vi "Eval.vi"(10 "String":string="1 + 1", 11 "NameSpace":variant) -> (3 "element":dbl)   [LabVIEW 2019, in "Eval.lvlib"]
uses:
  Library/Eval.lvlib
  <vilib>/Utility/Data Type/NI_Data Type.lvlib
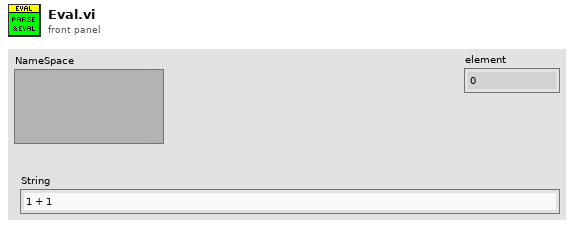
[diagram p1: front panel]
types:
  T1 = cluster{"Token":enum16{"ADD", "BITAND", "BITOR", "COMMA", "DIV", "Dnumeric", "EQUAL", "EXP", "FUNC", "GREATER", "GREATEREQ", "INumeric", "Identifier", "Ignore", "LESS", "LESSEQ", "LOGAND", "LOGOR", "LPAR", "LSHIFT", "MULT", "N/A", "RPAR", "RSHIFT", "SUB", "UADD", "USUB"}, "Priority":i32, "Type":enum16{"N/A", "GroupL", "GroupR", "Comma", "Operator", "Operand", "End"}, "Associtivity":enum16{"N/A", "L-R", "R-L"}, "GroupPair":i32}[]
  T2 = cluster{"NextTable":enum16{"#Init", "And", "Bin", "CompG", "CompL", "DNumeric", "INumeric", "Identifier", "Or", "Unreachable"}, "Actions":enum16{"Drop", "Hold", "Push"}, "Token":enum16{"ADD", "BITAND", "BITOR", "COMMA", "DIV", "Dnumeric", "EQUAL", "EXP", "FUNC", "GREATER", "GREATEREQ", "INumeric", "Identifier", "Ignore", "LESS", "LESSEQ", "LOGAND", "LOGOR", "LPAR", "LSHIFT", "MULT", "N/A", "RPAR", "RSHIFT", "SUB", "UADD", "USUB"}}[]
  T3 = cluster{"NextTable":enum16{"#Init", "And", "Bin", "CompG", "CompL", "DNumeric", "INumeric", "Identifier", "Or", "Unreachable"}, "Actions":enum16{"Drop", "Hold", "Push"}, "Token":enum16{"ADD", "BITAND", "BITOR", "COMMA", "DIV", "Dnumeric", "EQUAL", "EXP", "FUNC", "GREATER", "GREATEREQ", "INumeric", "Identifier", "Ignore", "LESS", "LESSEQ", "LOGAND", "LOGOR", "LPAR", "LSHIFT", "MULT", "N/A", "RPAR", "RSHIFT", "SUB", "UADD", "USUB"}}
  T4 = enum16{"ADD", "BITAND", "BITOR", "COMMA", "DIV", "Dnumeric", "EQUAL", "EXP", "FUNC", "GREATER", "GREATEREQ", "INumeric", "Identifier", "Ignore", "LESS", "LESSEQ", "LOGAND", "LOGOR", "LPAR", "LSHIFT", "MULT", "N/A", "RPAR", "RSHIFT", "SUB", "UADD", "USUB"}
  T5 = cluster{"Start":i32, "End":i32, "Token":enum16{"ADD", "BITAND", "BITOR", "COMMA", "DIV", "Dnumeric", "EQUAL", "EXP", "FUNC", "GREATER", "GREATEREQ", "INumeric", "Identifier", "Ignore", "LESS", "LESSEQ", "LOGAND", "LOGOR", "LPAR", "LSHIFT", "MULT", "N/A", "RPAR", "RSHIFT", "SUB", "UADD", "USUB"}}
  T6 = cluster{"Start":i32, "End":i32, "Token":enum16{"ADD", "BITAND", "BITOR", "COMMA", "DIV", "Dnumeric", "EQUAL", "EXP", "FUNC", "GREATER", "GREATEREQ", "INumeric", "Identifier", "Ignore", "LESS", "LESSEQ", "LOGAND", "LOGOR", "LPAR", "LSHIFT", "MULT", "N/A", "RPAR", "RSHIFT", "SUB", "UADD", "USUB"}}[]
  T7 = enum16{"#Init", "And", "Bin", "CompG", "CompL", "DNumeric", "INumeric", "Identifier", "Or", "Unreachable"}
  T8 = cluster{"Token":enum16{"ADD", "BITAND", "BITOR", "COMMA", "DIV", "Dnumeric", "EQUAL", "EXP", "FUNC", "GREATER", "GREATEREQ", "INumeric", "Identifier", "Ignore", "LESS", "LESSEQ", "LOGAND", "LOGOR", "LPAR", "LSHIFT", "MULT", "N/A", "RPAR", "RSHIFT", "SUB", "UADD", "USUB"}, "Priority":i32, "Type":enum16{"N/A", "GroupL", "GroupR", "Comma", "Operator", "Operand", "End"}, "Associtivity":enum16{"N/A", "L-R", "R-L"}, "GroupPair":i32}
  T9 = enum16{"N/A", "GroupL", "GroupR", "Comma", "Operator", "Operand", "End"}
  T10 = typedef "NI_Data Type.lvlib/Data Type.ctl" = enum8{"Invalid Type", "Void", "I8", "I16", "I32", "I64", "U8", "U16", "U32", "U64", "Single Float", "Double Float", "Extended Float", "Single Complex", "Double Complex", "Extended Complex", "Enum U8", "Enum U16", "Enum U32", "Enum U64", "Single Float With Unit", "Double Float With Unit", "Extended Float With Unit", "Single Complex with Unit", "Double Complex with Unit", "Extended Complex with Unit", "Boolean", "String", "Path", "Picture", "Tag", "Array", "Cluster", "Variant", "LV Variant", "Waveform", "Timestamp", "Digital Waveform", "Digital Data", "ExpressData", "Refnum", "External Data", "VI", "Poly VI", "LabVIEW Class Instance", "Fixed Point", "Set Collection", "Map Collection"}
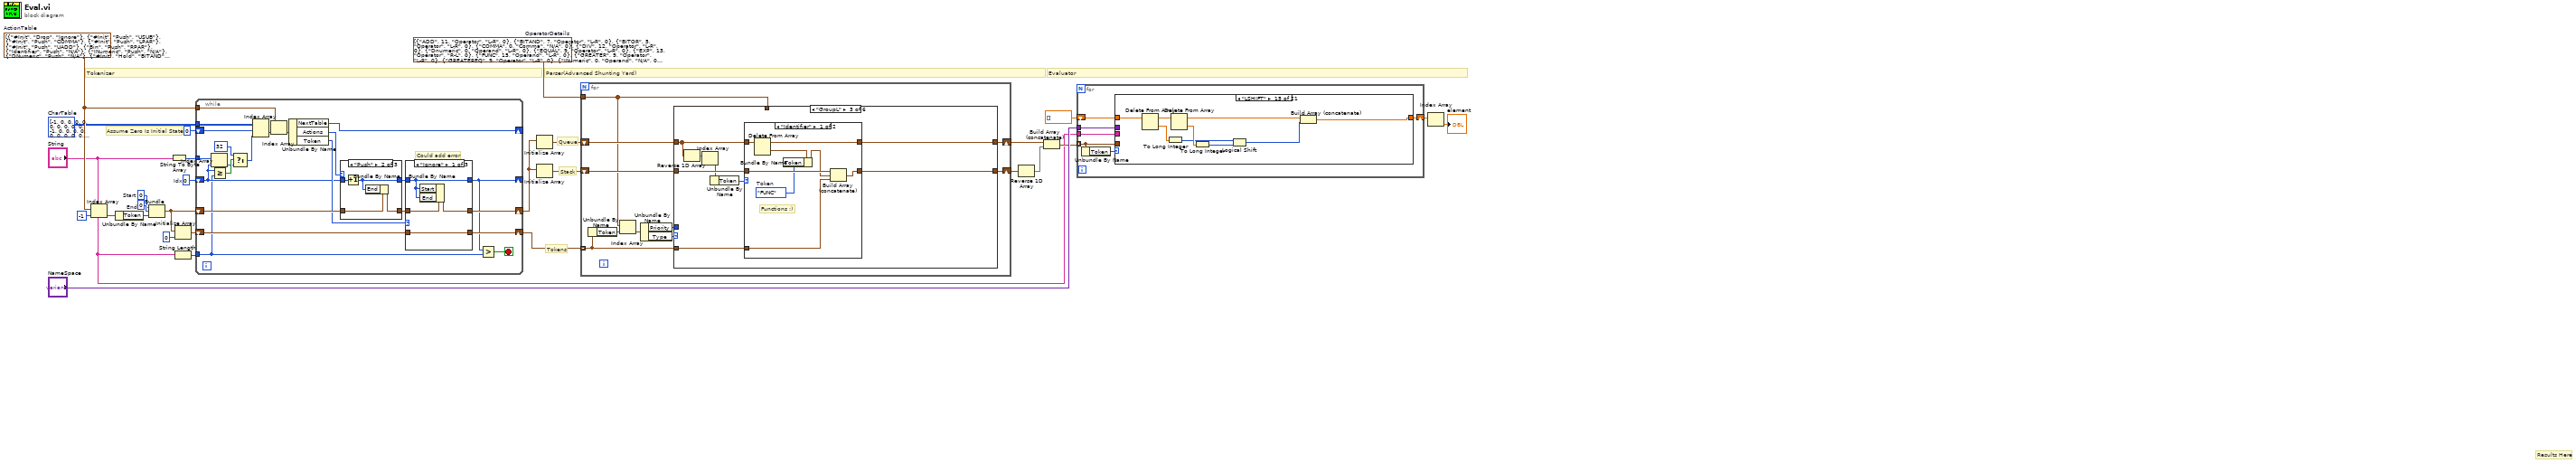
[diagram p0: block diagram]
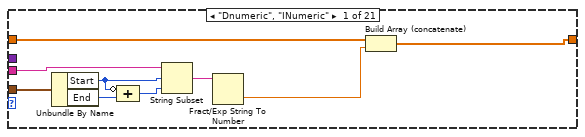
[diagram p2: hidden frame]
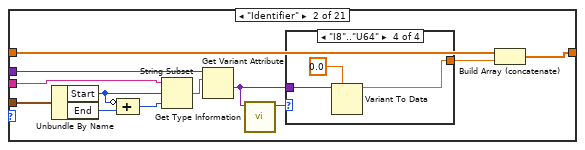
[diagram p3: hidden frame]
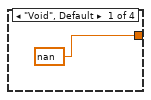
[diagram p4: hidden frame]
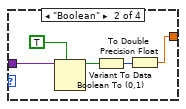
[diagram p5: hidden frame]
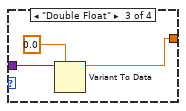
[diagram p6: hidden frame]
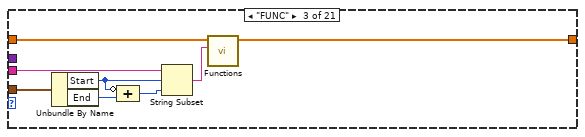
[diagram p7: hidden frame]
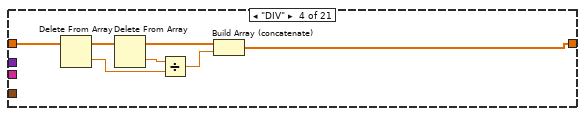
[diagram p8: hidden frame]
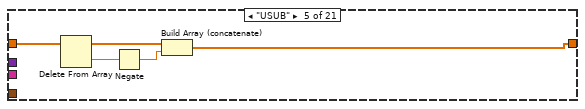
[diagram p9: hidden frame]
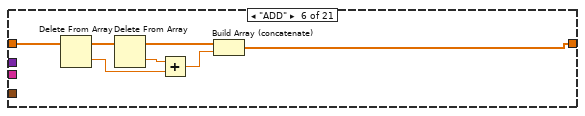
[diagram p10: hidden frame]
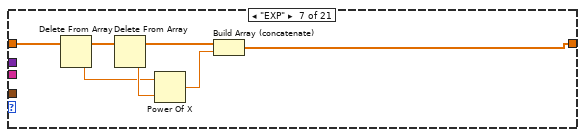
[diagram p11: hidden frame]
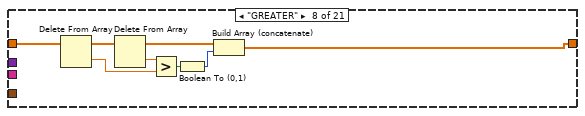
[diagram p12: hidden frame]
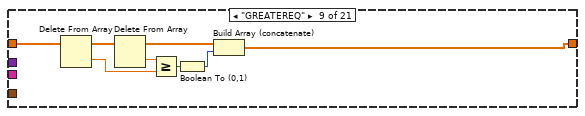
[diagram p13: hidden frame]
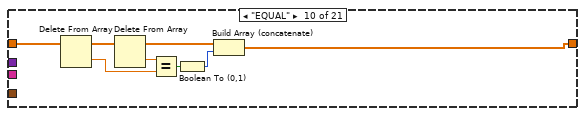
[diagram p14: hidden frame]
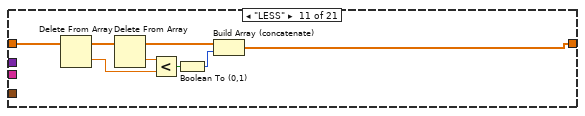
[diagram p15: hidden frame]
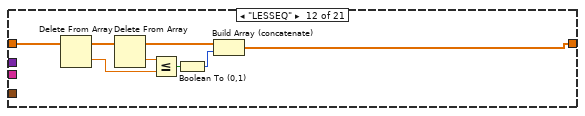
[diagram p16: hidden frame]
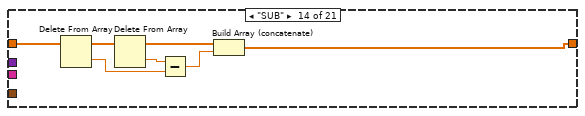
[diagram p18: hidden frame]
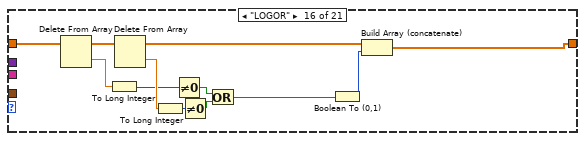
[diagram p19: hidden frame]
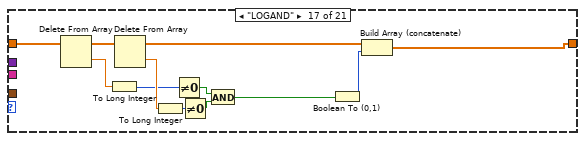
[diagram p20: hidden frame]
diagram:
  w3 = i32[][] [[-1, 0, 0, 0, 0, 0, 0, 0, 0, 0, -1, 0, 0, 0, 0, 0, 0, 0, 0, 0, 0, 0, 0, 0, 0, 0, 0, 0, 0, 0, 0, 0, 0, 0, 0, 0, 0, 0, 0, 0, 3, 5, 0, 4, 2, 1, 8, 0, 7, 7, 7, 7, 7, 7, 7, 7, 7, 7, 0, 0, 0, 0, 0, 0, 0, 6, 6, 6, 6, 6, 6, 6, 6, 6, 6, 6, 6, 6, 6, 6, 6, 6, 6, 6, 6, 6, 6, 6, 6, 6, 6, 0, 0, 0, 0, 6, 0, 6, 6, 6, 6, 6, 6, 6, 6, 6, 6, 6, 6, 6, 6, 6, 6, 6, 6, 6, 6, 6, 6, 6, 6, 6, 6, 0, 0, 0, 0, 0, 0, 0, 0, 0, 0, 0, 0, 0, 0, 0, 0, 0, 0, 0, 0, 0, 0, 0, 0, 0, 0, 0, 0, 0, 0, 0, 0, 0, 0, 0, 0, 0, 0, 0, 0, 0, 0, 0, 0, 0, 0, 0, 0, 0, 0, 0, 0, 0, 0, 0, 0, 0, 0, 0, 0, 0, 0, 0, 0, 0, 0, 0, 0, 0, 0, 0, 0, 0, 0, 0, 0, 0, 0, 0, 0, 0, 0, 0, 0, 0, 0, 0, 0, 0, 0, 0, 0, 0, 0, 0, 0, 0, 0, 0, 0, 0, 0, 0, 0, 0, 0, 0, 0, 0, 0, 0, 0, 0, 0, 0, 0, 0, 0, 0, 0, 0, 0, 0, 0, 0, 0, 0, 0, 0, 0, 0, 0], [-1, 9, 9, 9, 9, 9, 9, 9, 9, 9, -1, 9, 9, 9, 9, 9, 9, 9, 9, 9, 9, 9, 9, 9, 9, 9, 9, 9, 9, 9, 9, 9, 9, 9, 9, 9, 9, 9, 10, 9, 9, 9, 9, 9, 9, 9, 9, 9, 9, 9, 9, 9, 9, 9, 9, 9, 9, 9, 9, 9, 9, 9, 9, 9, 9, 9, 9, 9, 9, 9, 9, 9, 9, 9, 9, 9, 9, 9, 9, 9, 9, 9, 9, 9, 9, 9, 9, 9, 9, 9, 9, 9, 9, 9, 9, 9, 9, 9, 9, 9, 9, 9, 9, 9, 9, 9, 9, 9, 9, 9, 9, 9, 9, 9, 9, 9, 9, 9, 9, 9, 9, 9, 9, 9, 9, 9, 9, 9, 9, 9, 9, 9, 9, 9, 9, 9, 9, 9, 9, 9, 9, 9, 9, 9, 9, 9, 9, 9, 9, 9, 9, 9, 9, 9, 9, 9, 9, 9, 9, 9, 9, 9, 9, 9, 9, 9, 9, 9, 9, 9, 9, 9, 9, 9, 9, 9, 9, 9, 9, 9, 9, 9, 9, 9, 9, 9, 9, 9, 9, 9, 9, 9, 9, 9, 9, 9, 9, 9, 9, 9, 9, 9, 9, 9, 9, 9, 9, 9, 9, 9, 9, 9, 9, 9, 9, 9, 9, 9, 9, 9, 9, 9, 9, 9, 9, 9, 9, 9, 9, 9, 9, 9, 9, 9, 9, 9, 9, 9, 9, 9, 9, 9, 9, 9, 9, 9, 9, 9, 9, 9, 9, 9, 9, 9, 9], [-1, 11, 11, 11, 11, 11, 11, 11, 11, 11, -1, 11, 11, 11, 11, 11, 11, 11, 11, 11, 11, 11, 11, 11, 11, 11, 11, 11, 11, 11, 11, 11, 11, 11, 11, 11, 11, 11, 24, 11, 16, 20, 15, 17, 14, 13, 27, 12, 26, 26, 26, 26, 26, 26, 26, 26, 26, 26, 11, 11, 22, 18, 21, 11, 11, 25, 25, 25, 25, 25, 25, 25, 25, 25, 25, 25, 25, 25, 25, 25, 25, 25, 25, 25, 25, 25, 25, 25, 25, 25, 25, 11, 11, 11, 19, 25, 11, 25, 25, 25, 25, 25, 25, 25, 25, 25, 25, 25, 25, 25, 25, 25, 25, 25, 25, 25, 25, 25, 25, 25, 25, 25, 25, 11, 23, 11, 11, 11, 11, 11, 11, 11, 11, 11, 11, 11, 11, 11, 11, 11, 11, 11, 11, 11, 11, 11, 11, 11, 11, 11, 11, 11, 11, 11, 11, 11, 11, 11, 11, 11, 11, 11, 11, 11, 11, 11, 11, 11, 11, 11, 11, 11, 11, 11, 11, 11, 11, 11, 11, 11, 11, 11, 11, 11, 11, 11, 11, 11, 11, 11, 11, 11, 11, 11, 11, 11, 11, 11, 11, 11, 11, 11, 11, 11, 11, 11, 11, 11, 11, 11, 11, 11, 11, 11, 11, 11, 11, 11, 11, 11, 11, 11, 11, 11, 11, 11, 11, 11, 11, 11, 11, 11, 11, 11, 11, 11, 11, 11, 11, 11, 11, 11, 11, 11, 11, 11, 11, 11, 11, 11, 11, 11, 11, 11, 11], [-1, 28, 28, 28, 28, 28, 28, 28, 28, 28, -1, 28, 28, 28, 28, 28, 28, 28, 28, 28, 28, 28, 28, 28, 28, 28, 28, 28, 28, 28, 28, 28, 28, 28, 28, 28, 28, 28, 28, 28, 28, 28, 28, 28, 28, 28, 28, 28, 28, 28, 28, 28, 28, 28, 28, 28, 28, 28, 28, 28, 28, 29, 30, 28, 28, 28, 28, 28, 28, 28, 28, 28, 28, 28, 28, 28, 28, 28, 28, 28, 28, 28, 28, 28, 28, 28, 28, 28, 28, 28, 28, 28, 28, 28, 28, 28, 28, 28, 28, 28, 28, 28, 28, 28, 28, 28, 28, 28, 28, 28, 28, 28, 28, 28, 28, 28, 28, 28, 28, 28, 28, 28, 28, 28, 28, 28, 28, 28, 28, 28, 28, 28, 28, 28, 28, 28, 28, 28, 28, 28, 28, 28, 28, 28, 28, 28, 28, 28, 28, 28, 28, 28, 28, 28, 28, 28, 28, 28, 28, 28, 28, 28, 28, 28, 28, 28, 28, 28, 28, 28, 28, 28, 28, 28, 28, 28, 28, 28, 28, 28, 28, 28, 28, 28, 28, 28, 28, 28, 28, 28, 28, 28, 28, 28, 28, 28, 28, 28, 28, 28, 28, 28, 28, 28, 28, 28, 28, 28, 28, 28, 28, 28, 28, 28, 28, 28, 28, 28, 28, 28, 28, 28, 28, 28, 28, 28, 28, 28, 28, 28, 28, 28, 28, 28, 28, 28, 28, 28, 28, 28, 28, 28, 28, 28, 28, 28, 28, 28, 28, 28, 28, 28, 28, 28, 28], [-1, 31, 31, 31, 31, 31, 31, 31, 31, 31, -1, 31, 31, 31, 31, 31, 31, 31, 31, 31, 31, 31, 31, 31, 31, 31, 31, 31, 31, 31, 31, 31, 31, 31, 31, 31, 31, 31, 31, 31, 31, 31, 31, 31, 31, 31, 31, 31, 31, 31, 31, 31, 31, 31, 31, 31, 31, 31, 31, 31, 33, 32, 31, 31, 31, 31, 31, 31, 31, 31, 31, 31, 31, 31, 31, 31, 31, 31, 31, 31, 31, 31, 31, 31, 31, 31, 31, 31, 31, 31, 31, 31, 31, 31, 31, 31, 31, 31, 31, 31, 31, 31, 31, 31, 31, 31, 31, 31, 31, 31, 31, 31, 31, 31, 31, 31, 31, 31, 31, 31, 31, 31, 31, 31, 31, 31, 31, 31, 31, 31, 31, 31, 31, 31, 31, 31, 31, 31, 31, 31, 31, 31, 31, 31, 31, 31, 31, 31, 31, 31, 31, 31, 31, 31, 31, 31, 31, 31, 31, 31, 31, 31, 31, 31, 31, 31, 31, 31, 31, 31, 31, 31, 31, 31, 31, 31, 31, 31, 31, 31, 31, 31, 31, 31, 31, 31, 31, 31, 31, 31, 31, 31, 31, 31, 31, 31, 31, 31, 31, 31, 31, 31, 31, 31, 31, 31, 31, 31, 31, 31, 31, 31, 31, 31, 31, 31, 31, 31, 31, 31, 31, 31, 31, 31, 31, 31, 31, 31, 31, 31, 31, 31, 31, 31, 31, 31, 31, 31, 31, 31, 31, 31, 31, 31, 31, 31, 31, 31, 31, 31, 31, 31, 31, 31, 31], [-1, 34, 34, 34, 34, 34, 34, 34, 34, 34, -1, 34, 34, 34, 34, 34, 34, 34, 34, 34, 34, 34, 34, 34, 34, 34, 34, 34, 34, 34, 34, 34, 34, 34, 34, 34, 34, 34, 34, 34, 34, 34, 34, 34, 34, 34, 34, 34, 35, 35, 35, 35, 35, 35, 35, 35, 35, 35, 34, 34, 34, 34, 34, 34, 34, 34, 34, 34, 34, 34, 34, 34, 34, 34, 34, 34, 34, 34, 34, 34, 34, 34, 34, 34, 34, 34, 34, 34, 34, 34, 34, 34, 34, 34, 34, 34, 34, 34, 34, 34, 34, 34, 34, 34, 34, 34, 34, 34, 34, 34, 34, 34, 34, 34, 34, 34, 34, 34, 34, 34, 34, 34, 34, 34, 34, 34, 34, 34, 34, 34, 34, 34, 34, 34, 34, 34, 34, 34, 34, 34, 34, 34, 34, 34, 34, 34, 34, 34, 34, 34, 34, 34, 34, 34, 34, 34, 34, 34, 34, 34, 34, 34, 34, 34, 34, 34, 34, 34, 34, 34, 34, 34, 34, 34, 34, 34, 34, 34, 34, 34, 34, 34, 34, 34, 34, 34, 34, 34, 34, 34, 34, 34, 34, 34, 34, 34, 34, 34, 34, 34, 34, 34, 34, 34, 34, 34, 34, 34, 34, 34, 34, 34, 34, 34, 34, 34, 34, 34, 34, 34, 34, 34, 34, 34, 34, 34, 34, 34, 34, 34, 34, 34, 34, 34, 34, 34, 34, 34, 34, 34, 34, 34, 34, 34, 34, 34, 34, 34, 34, 34, 34, 34, 34, 34, 34], [-1, 36, 36, 36, 36, 36, 36, 36, 36, 36, -1, 36, 36, 36, 36, 36, 36, 36, 36, 36, 36, 36, 36, 36, 36, 36, 36, 36, 36, 36, 36, 36, 36, 36, 36, 36, 36, 36, 36, 36, 36, 36, 36, 36, 36, 36, 38, 36, 37, 37, 37, 37, 37, 37, 37, 37, 37, 37, 36, 36, 36, 36, 36, 36, 36, 36, 36, 36, 36, 36, 36, 36, 36, 36, 36, 36, 36, 36, 36, 36, 36, 36, 36, 36, 36, 36, 36, 36, 36, 36, 36, 36, 36, 36, 36, 36, 36, 36, 36, 36, 36, 36, 36, 36, 36, 36, 36, 36, 36, 36, 36, 36, 36, 36, 36, 36, 36, 36, 36, 36, 36, 36, 36, 36, 36, 36, 36, 36, 36, 36, 36, 36, 36, 36, 36, 36, 36, 36, 36, 36, 36, 36, 36, 36, 36, 36, 36, 36, 36, 36, 36, 36, 36, 36, 36, 36, 36, 36, 36, 36, 36, 36, 36, 36, 36, 36, 36, 36, 36, 36, 36, 36, 36, 36, 36, 36, 36, 36, 36, 36, 36, 36, 36, 36, 36, 36, 36, 36, 36, 36, 36, 36, 36, 36, 36, 36, 36, 36, 36, 36, 36, 36, 36, 36, 36, 36, 36, 36, 36, 36, 36, 36, 36, 36, 36, 36, 36, 36, 36, 36, 36, 36, 36, 36, 36, 36, 36, 36, 36, 36, 36, 36, 36, 36, 36, 36, 36, 36, 36, 36, 36, 36, 36, 36, 36, 36, 36, 36, 36, 36, 36, 36, 36, 36, 36], [-1, 39, 39, 39, 39, 39, 39, 39, 39, 39, -1, 39, 39, 39, 39, 39, 39, 39, 39, 39, 39, 39, 39, 39, 39, 39, 39, 39, 39, 39, 39, 39, 39, 39, 39, 39, 39, 39, 39, 39, 39, 39, 39, 39, 39, 39, 39, 39, 40, 40, 40, 40, 40, 40, 40, 40, 40, 40, 39, 39, 39, 39, 39, 39, 39, 40, 40, 40, 40, 40, 40, 40, 40, 40, 40, 40, 40, 40, 40, 40, 40, 40, 40, 40, 40, 40, 40, 40, 40, 40, 40, 39, 39, 39, 39, 40, 39, 40, 40, 40, 40, 40, 40, 40, 40, 40, 40, 40, 40, 40, 40, 40, 40, 40, 40, 40, 40, 40, 40, 40, 40, 40, 40, 39, 39, 39, 39, 39, 39, 39, 39, 39, 39, 39, 39, 39, 39, 39, 39, 39, 39, 39, 39, 39, 39, 39, 39, 39, 39, 39, 39, 39, 39, 39, 39, 39, 39, 39, 39, 39, 39, 39, 39, 39, 39, 39, 39, 39, 39, 39, 39, 39, 39, 39, 39, 39, 39, 39, 39, 39, 39, 39, 39, 39, 39, 39, 39, 39, 39, 39, 39, 39, 39, 39, 39, 39, 39, 39, 39, 39, 39, 39, 39, 39, 39, 39, 39, 39, 39, 39, 39, 39, 39, 39, 39, 39, 39, 39, 39, 39, 39, 39, 39, 39, 39, 39, 39, 39, 39, 39, 39, 39, 39, 39, 39, 39, 39, 39, 39, 39, 39, 39, 39, 39, 39, 39, 39, 39, 39, 39, 39, 39, 39, 39, 39], [-1, 41, 41, 41, 41, 41, 41, 41, 41, 41, -1, 41, 41, 41, 41, 41, 41, 41, 41, 41, 41, 41, 41, 41, 41, 41, 41, 41, 41, 41, 41, 41, 41, 41, 41, 41, 41, 41, 41, 41, 41, 41, 41, 41, 41, 41, 41, 41, 41, 41, 41, 41, 41, 41, 41, 41, 41, 41, 41, 41, 41, 41, 41, 41, 41, 41, 41, 41, 41, 41, 41, 41, 41, 41, 41, 41, 41, 41, 41, 41, 41, 41, 41, 41, 41, 41, 41, 41, 41, 41, 41, 41, 41, 41, 41, 41, 41, 41, 41, 41, 41, 41, 41, 41, 41, 41, 41, 41, 41, 41, 41, 41, 41, 41, 41, 41, 41, 41, 41, 41, 41, 41, 41, 41, 42, 41, 41, 41, 41, 41, 41, 41, 41, 41, 41, 41, 41, 41, 41, 41, 41, 41, 41, 41, 41, 41, 41, 41, 41, 41, 41, 41, 41, 41, 41, 41, 41, 41, 41, 41, 41, 41, 41, 41, 41, 41, 41, 41, 41, 41, 41, 41, 41, 41, 41, 41, 41, 41, 41, 41, 41, 41, 41, 41, 41, 41, 41, 41, 41, 41, 41, 41, 41, 41, 41, 41, 41, 41, 41, 41, 41, 41, 41, 41, 41, 41, 41, 41, 41, 41, 41, 41, 41, 41, 41, 41, 41, 41, 41, 41, 41, 41, 41, 41, 41, 41, 41, 41, 41, 41, 41, 41, 41, 41, 41, 41, 41, 41, 41, 41, 41, 41, 41, 41, 41, 41, 41, 41, 41, 41, 41, 41, 41, 41, 41], [-1, 43, 43, 43, 43, 43, 43, 43, 43, 43, -1, 43, 43, 43, 43, 43, 43, 43, 43, 43, 43, 43, 43, 43, 43, 43, 43, 43, 43, 43, 43, 43, 43, 43, 43, 43, 43, 43, 43, 43, 43, 43, 43, 43, 43, 43, 43, 43, 43, 43, 43, 43, 43, 43, 43, 43, 43, 43, 43, 43, 43, 43, 43, 43, 43, 43, 43, 43, 43, 43, 43, 43, 43, 43, 43, 43, 43, 43, 43, 43, 43, 43, 43, 43, 43, 43, 43, 43, 43, 43, 43, 43, 43, 43, 43, 43, 43, 43, 43, 43, 43, 43, 43, 43, 43, 43, 43, 43, 43, 43, 43, 43, 43, 43, 43, 43, 43, 43, 43, 43, 43, 43, 43, 43, 43, 43, 43, 43, 43, 43, 43, 43, 43, 43, 43, 43, 43, 43, 43, 43, 43, 43, 43, 43, 43, 43, 43, 43, 43, 43, 43, 43, 43, 43, 43, 43, 43, 43, 43, 43, 43, 43, 43, 43, 43, 43, 43, 43, 43, 43, 43, 43, 43, 43, 43, 43, 43, 43, 43, 43, 43, 43, 43, 43, 43, 43, 43, 43, 43, 43, 43, 43, 43, 43, 43, 43, 43, 43, 43, 43, 43, 43, 43, 43, 43, 43, 43, 43, 43, 43, 43, 43, 43, 43, 43, 43, 43, 43, 43, 43, 43, 43, 43, 43, 43, 43, 43, 43, 43, 43, 43, 43, 43, 43, 43, 43, 43, 43, 43, 43, 43, 43, 43, 43, 43, 43, 43, 43, 43, 43, 43, 43, 43, 43, 43]]  # CharTable
  w9 = T1 [{"Token"=enum."ADD", "Priority"=11, "Type"=enum."Operator", "Associtivity"=enum."L-R", "GroupPair"=0}, {"Token"=enum."BITAND", "Priority"=7, "Type"=enum."Operator", "Associtivity"=enum."L-R", "GroupPair"=0}, {"Token"=enum."BITOR", "Priority"=5, "Type"=enum."Operator", "Associtivity"=enum."L-R", "GroupPair"=0}, {"Token"=enum."COMMA", "Priority"=0, "Type"=enum."Comma", "Associtivity"=enum."N/A", "GroupPair"=0}, {"Token"=enum."DIV", "Priority"=12, "Type"=enum."Operator", "Associtivity"=enum."L-R", "GroupPair"=0}, {"Token"=enum."Dnumeric", "Priority"=0, "Type"=enum."Operand", "Associtivity"=enum."L-R", "GroupPair"=0}, {"Token"=enum."EQUAL", "Priority"=9, "Type"=enum."Operator", "Associtivity"=enum."L-R", "GroupPair"=0}, {"Token"=enum."EXP", "Priority"=13, "Type"=enum."Operator", "Associtivity"=enum."R-L", "GroupPair"=0}, {"Token"=enum."FUNC", "Priority"=15, "Type"=enum."Operand", "Associtivity"=enum."L-R", "GroupPair"=0}, {"Token"=enum."GREATER", "Priority"=9, "Type"=enum."Operator", "Associtivity"=enum."L-R", "GroupPair"=0}, {"Token"=enum."GREATEREQ", "Priority"=9, "Type"=enum."Operator", "Associtivity"=enum."L-R", "GroupPair"=0}, {"Token"=enum."INumeric", "Priority"=0, "Type"=enum."Operand", "Associtivity"=enum."N/A", "GroupPair"=0}, {"Token"=enum."Identifier", "Priority"=0, "Type"=enum."Operand", "Associtivity"=enum."N/A", "GroupPair"=0}, {"Token"=enum."Ignore", "Priority"=0, "Type"=enum."N/A", "Associtivity"=enum."N/A", "GroupPair"=0}, {"Token"=enum."LESS", "Priority"=9, "Type"=enum."Operator", "Associtivity"=enum."L-R", "GroupPair"=0}, {"Token"=enum."LESSEQ", "Priority"=9, "Type"=enum."Operator", "Associtivity"=enum."L-R", "GroupPair"=0}, {"Token"=enum."LOGAND", "Priority"=4, "Type"=enum."Operator", "Associtivity"=enum."L-R", "GroupPair"=0}, {"Token"=enum."LOGOR", "Priority"=3, "Type"=enum."Operator", "Associtivity"=enum."L-R", "GroupPair"=0}, {"Token"=enum."LPAR", "Priority"=0, "Type"=enum."GroupL", "Associtivity"=enum."N/A", "GroupPair"=1}, {"Token"=enum."LSHIFT", "Priority"=10, "Type"=enum."Operator", "Associtivity"=enum."L-R", "GroupPair"=0}, {"Token"=enum."MULT", "Priority"=12, "Type"=enum."Operator", "Associtivity"=enum."N/A", "GroupPair"=0}, {"Token"=enum."N/A", "Priority"=0, "Type"=enum."Operand", "Associtivity"=enum."N/A", "GroupPair"=0}, {"Token"=enum."RPAR", "Priority"=0, "Type"=enum."GroupR", "Associtivity"=enum."N/A", "GroupPair"=1}, {"Token"=enum."RSHIFT", "Priority"=10, "Type"=enum."Operator", "Associtivity"=enum."L-R", "GroupPair"=0}, {"Token"=enum."SUB", "Priority"=11, "Type"=enum."Operator", "Associtivity"=enum."L-R", "GroupPair"=0}, {"Token"=enum."UADD", "Priority"=14, "Type"=enum."Operator", "Associtivity"=enum."R-L", "GroupPair"=0}, {"Token"=enum."USUB", "Priority"=14, "Type"=enum."Operator", "Associtivity"=enum."R-L", "GroupPair"=0}]  # OperatorDetails
  w16 = T2 [{"NextTable"=enum."#Init", "Actions"=enum."Drop", "Token"=enum."Ignore"}, {"NextTable"=enum."#Init", "Actions"=enum."Push", "Token"=enum."USUB"}, {"NextTable"=enum."#Init", "Actions"=enum."Push", "Token"=enum."COMMA"}, {"NextTable"=enum."#Init", "Actions"=enum."Push", "Token"=enum."LPAR"}, {"NextTable"=enum."#Init", "Actions"=enum."Push", "Token"=enum."UADD"}, {"NextTable"=enum."Bin", "Actions"=enum."Push", "Token"=enum."RPAR"}, {"NextTable"=enum."Identifier", "Actions"=enum."Push", "Token"=enum."N/A"}, {"NextTable"=enum."INumeric", "Actions"=enum."Push", "Token"=enum."N/A"}, {"NextTable"=enum."DNumeric", "Actions"=enum."Push", "Token"=enum."N/A"}, {"NextTable"=enum."#Init", "Actions"=enum."Hold", "Token"=enum."BITAND"}, {"NextTable"=enum."#Init", "Actions"=enum."Push", "Token"=enum."LOGAND"}, {"NextTable"=enum."Bin", "Actions"=enum."Drop", "Token"=enum."Ignore"}, {"NextTable"=enum."#Init", "Actions"=enum."Push", "Token"=enum."DIV"}, {"NextTable"=enum."#Init", "Actions"=enum."Push", "Token"=enum."SUB"}, {"NextTable"=enum."#Init", "Actions"=enum."Push", "Token"=enum."COMMA"}, {"NextTable"=enum."#Init", "Actions"=enum."Push", "Token"=enum."MULT"}, {"NextTable"=enum."#Init", "Actions"=enum."Push", "Token"=enum."LPAR"}, {"NextTable"=enum."#Init", "Actions"=enum."Push", "Token"=enum."ADD"}, {"NextTable"=enum."#Init", "Actions"=enum."Push", "Token"=enum."EQUAL"}, {"NextTable"=enum."#Init", "Actions"=enum."Push", "Token"=enum."EXP"}, {"NextTable"=enum."Bin", "Actions"=enum."Push", "Token"=enum."RPAR"}, {"NextTable"=enum."CompG", "Actions"=enum."Push", "Token"=enum."N/A"}, {"NextTable"=enum."CompL", "Actions"=enum."Push", "Token"=enum."N/A"}, {"NextTable"=enum."Or", "Actions"=enum."Push", "Token"=enum."N/A"}, {"NextTable"=enum."And", "Actions"=enum."Push", "Token"=enum."N/A"}, {"NextTable"=enum."Identifier", "Actions"=enum."Push", "Token"=enum."N/A"}, {"NextTable"=enum."INumeric", "Actions"=enum."Push", "Token"=enum."N/A"}, {"NextTable"=enum."DNumeric", "Actions"=enum."Push", "Token"=enum."N/A"}, {"NextTable"=enum."#Init", "Actions"=enum."Hold", "Token"=enum."GREATER"}, {"NextTable"=enum."#Init", "Actions"=enum."Push", "Token"=enum."GREATEREQ"}, {"NextTable"=enum."#Init", "Actions"=enum."Push", "Token"=enum."RSHIFT"}, {"NextTable"=enum."#Init", "Actions"=enum."Hold", "Token"=enum."LESS"}, {"NextTable"=enum."#Init", "Actions"=enum."Push", "Token"=enum."LESSEQ"}, {"NextTable"=enum."#Init", "Actions"=enum."Push", "Token"=enum."LSHIFT"}, {"NextTable"=enum."Bin", "Actions"=enum."Hold", "Token"=enum."Dnumeric"}, {"NextTable"=enum."DNumeric", "Actions"=enum."Push", "Token"=enum."N/A"}, {"NextTable"=enum."Bin", "Actions"=enum."Hold", "Token"=enum."INumeric"}, {"NextTable"=enum."INumeric", "Actions"=enum."Push", "Token"=enum."N/A"}, {"NextTable"=enum."DNumeric", "Actions"=enum."Push", "Token"=enum."N/A"}, {"NextTable"=enum."Bin", "Actions"=enum."Hold", "Token"=enum."Identifier"}, {"NextTable"=enum."Identifier", "Actions"=enum."Push", "Token"=enum."N/A"}, {"NextTable"=enum."#Init", "Actions"=enum."Hold", "Token"=enum."BITOR"}, {"NextTable"=enum."#Init", "Actions"=enum."Push", "Token"=enum."LOGOR"}, {"NextTable"=enum."#Init", "Actions"=enum."Hold", "Token"=enum."FUNC"}]  # ActionTable
  w24 = 0  # End
  w23 = 0  # Start
  w21 = 0  # Idx
  # "Tokens"
  # "Queue"
  # "Stack"
  # "Assume Zero Is Initial State"
  # "Evaluator"
  # "Parser(Advanced Shunting Yard)"
  # "Tokenizer"
  # "Results Here"
  n1 = Index Array(array=w16, index=-1) -> (element=w14:T3)
  n2 = Unbundle By Name(w14) -> ("Token"=w13:T4)
  n3 = Bundle("Start"=w23, "End"=w24, "Token"=w13) -> (w25:T5)  [unwired: 1 in]
  n4 = String To Byte Array(string="String") -> (unsigned byte array=w22:u8[])
  n5 = Initialize Array(w25, 0 ("dimension size")) -> (w27:T6)
  n6 = String Length(string="String") -> (length=w2:i32)
  n7 = while {
    shift-right: [w48] -> _
    shift-left: u16 0 -> [w51]
    tunnel: w22 -> [w50]
    shift-right: [w41] -> w19
    shift-left: w25 -> [w46]
    shift-right: [w45] -> w12
    shift-left: w27 -> [w44]
    shift-right: [w39] -> _
    shift-left: w21 -> [w37]
    tunnel: w2 -> [w36]
    tunnel: w16 -> [w30]
    tunnel: w3 -> [w29]
    stop <- w31 stop-if-true
    # "Could add error"
    n8 = Index Array(array=w50, index=w37) -> (element=w33:u8)
    n9 = Greater Or Equal?(x=w37, y=w36) -> (x >= y?=w35:bool)
    n10 = Select(t=u8 32, s=w35, f=w33) -> (s? t:f=w32:u8)
    n11 = Index Array(array=w29, index (row)=w51, index (col)=w32) -> (element=w49:i32)
    n12 = Index Array(array=w30, index=w49) -> (element=w38:T3)
    n13 = Unbundle By Name(w38) -> ("NextTable"=w48:T7, "Actions"=w47:enum16{"Drop", "Hold", "Push"}, "Token"=w42:T4)
    n14 = case shown="\"Push\"" w47 {
      tunnel: w37 -> [w68 w72 w74]
      tunnel: w46 -> [w69 w73 w75]
      tunnel: [w66 w70 w74] -> w40
      tunnel: [w67 w71 w75] -> w43
      frame "Drop", Default {
        n15 = Increment(x=w68) -> (x+1=w66:i32)
        n16 = Bundle By Name(cluster=w69, "Start"=w66, "End"=w66) -> (w67:T5)
      }
      frame "Push" {
        n17 = Increment(x=w72) -> (x+1=w70:i32)
        n18 = Bundle By Name(cluster=w73, "End"=w70) -> (w71:T5)
      }
      frame "Hold" {
      }
    }
    n19 = case shown="\"Ignore\"" w42 {
      selector: w42 -> [_ w56 _]
      tunnel: w44 -> [w52 w60 w65]
      tunnel: [w52 w62 w65] -> w45
      tunnel: w43 -> [w55 w59 w63]
      tunnel: [w54 w58 w63] -> w41
      tunnel: w40 -> [w53 w57 w64]
      tunnel: [w53 w57 w64] -> w39
      frame "Ignore" {
        n20 = Bundle By Name(cluster=w55, "Start"=w53, "End"=w53) -> (w54:T5)
      }
      frame Default {
        n21 = Bundle By Name(cluster=w59, "Token"=w56) -> (w61:T5)
        n22 = Bundle By Name(cluster=w59, "Start"=w57, "End"=w57) -> (w58:T5)
        n23 = Build Array (concatenate)(w60, w61) -> (w62:T6)
      }
      frame "N/A" {
      }
    }
    n24 = Greater?(x=w39, y=w36) -> (0:w31:bool)
  }
  n25 = Initialize Array(w19) -> (w20:T6)  [unwired: 1 in]
  n26 = Initialize Array(w19) -> (w18:T6)  [unwired: 1 in]
  n27 = for {
    tunnel: w12 -> [w76] mode=indexing
    shift-right: [w83] -> w11
    shift-left: w20 -> [w85]
    shift-right: [w82] -> w10
    shift-left: w18 -> [w84]
    tunnel: w9 -> [w81]
    n28 = Unbundle By Name(w76) -> ("Token"=w80:T4)
    n29 = Index Array(array=w81, index=w80) -> (element=w79:T8)
    n30 = Unbundle By Name(w79) -> ("Priority"=w77:i32, "Type"=w78:T9)
    n31 = case shown="\"GroupL\"" w78 {
      tunnel: w85 -> [w87 w96 w142 w163 w190 w217]
      tunnel: w84 -> [w86 w89 w148 w165 w192 w216]
      tunnel: [w87 w95 w144 w162 w189 w215] -> w83
      tunnel: [w86 w93 w147 w164 w191 w216] -> w82
      tunnel: w76 -> [_ w92 w146 _ _ w214]
      tunnel: w81 -> [_ w91 _ w161 w188 _]
      tunnel: w77 -> [_ w90 _ _ _ _]
      frame Default {
      }
      frame "Operator" {
        n32 = Empty Array?(array=w89) -> (empty?=w88:bool)
        n33 = case shown="False" w88 {
          tunnel: w96 -> [w102 w140]
          tunnel: [w101 w140] -> w95
          tunnel: [w100 w139] -> w94
          tunnel: w89 -> [w99 w139]
          tunnel: w91 -> [w98 _]
          tunnel: w90 -> [w97 _]
          frame False {
            n34 = while {
              shift-right: [w117] -> w100
              shift-left: w99 -> [w103]
              shift-right: [w116] -> w101
              shift-left: w102 -> [w115]
              tunnel: w98 -> [w111]
              tunnel: w97 -> [w105]
              stop <- w114 continue-if-true
              n35 = Reverse 1D Array(array=w103) -> (reversed array=w110:T6)
              n36 = Index Array(array=w110) -> (element=w113:T5)  [unwired: 1 in]
              n37 = Unbundle By Name(w113) -> ("Token"=w109:T4)
              n38 = Index Array(array=w111, index=w109) -> (element=w112:T8)
              n39 = Unbundle By Name(w112) -> ("Type"=w108:T9, "Associtivity"=w107:enum16{"N/A", "L-R", "R-L"}, "Priority"=w106:i32)
              n40 = case shown="Default" w108 {
                tunnel: w107 -> [w121 _]
                tunnel: w106 -> [w120 _]
                tunnel: w105 -> [w119 _]
                tunnel: [w118 FALSE ("x != y?")] -> w104
                frame Default {
                  n41 = case shown="\"L-R\"" w121 {
                    tunnel: w120 -> [w124 w127]
                    tunnel: w119 -> [w123 w126]
                    tunnel: [w122 w125] -> w118
                    frame Default {
                      n42 = Greater?(x=w124, y=w123) -> (0:w122:bool)
                    }
                    frame "L-R" {
                      n43 = Greater Or Equal?(x=w127, y=w126) -> (x >= y?=w125:bool)
                    }
                  }
                }
                frame "GroupL" {
                }
              }
              n44 = case shown="True" w104 {
                selector: w104 -> [w129 _]
                tunnel: [w130 w134] -> w117
                tunnel: w103 -> [w130 w137]
                tunnel: [w131 w136] -> w116
                tunnel: w115 -> [w131 w138]
                tunnel: [w129 w132] -> w114
                frame False {
                }
                frame True {
                  n45 = Delete From Array(array=w137) -> (deleted portion=w135:T5, array with subset deleted=w134:T6)  [unwired: 2 in]
                  n46 = Empty Array?(array=w134) -> (empty?=w133:bool)
                  n47 = Build Array (concatenate)(w138, w135) -> (w136:T6)
                  n48 = Not(x=w133) -> (.not. x?=w132:bool)
                }
              }
            }
          }
          frame True {
            # "No need to look at the stack if its empty\nJust an optimization"
          }
        }
        n49 = Build Array (concatenate)(w94, w92) -> (w93:T6)
      }
      frame "GroupL" {
        n50 = Reverse 1D Array(array=w142) -> (reversed array=w143:T6)
        n51 = Index Array(array=w143) -> (element=w145:T5)  [unwired: 1 in]
        n52 = Unbundle By Name(w145) -> ("Token"=w141:T4)
        n53 = case shown="\"Identifier\"" w141 {
          tunnel: w148 -> [w156 w160]
          tunnel: [w155 w159] -> w147
          tunnel: w146 -> [w152 w158]
          tunnel: [w153 w157] -> w144
          tunnel: w142 -> [w154 w157]
          frame "Identifier" {
            w149 = T4."FUNC"  # Token
            # "Functions :)"
            n54 = Delete From Array(array=w154) -> (deleted portion=w151:T5, array with subset deleted=w153:T6)  [unwired: 2 in]
            n55 = Bundle By Name(cluster=w151, "Token"=w149) -> (w150:T5)
            n56 = Build Array (concatenate)(w156, w150, w152) -> (w155:T6)
          }
          frame Default {
            n57 = Build Array (concatenate)(w160, w158) -> (w159:T6)
          }
        }
      }
      frame "GroupR" {
        n58 = while {
          shift-right: [w169] -> w164
          shift-left: w165 -> [w166]
          shift-right: [w178] -> w162
          shift-left: w163 -> [w177]
          tunnel: w161 -> [w172]
          stop <- w168 stop-if-true
          n59 = Reverse 1D Array(array=w166) -> (reversed array=w174:T6)
          n60 = Index Array(array=w174) -> (element=w176:T5)  [unwired: 1 in]
          n61 = Unbundle By Name(w176) -> ("Token"=w173:T4)
          n62 = Index Array(array=w172, index=w173) -> (element=w171:T8)
          n63 = Unbundle By Name(w171) -> ("Type"=w170:T9)
          n64 = case shown="Default" w170 {
            tunnel: [w180 w187] -> w178
            tunnel: w177 -> [w181 w187]
            tunnel: [w182 w184] -> w169
            tunnel: w166 -> [w183 w185]
            tunnel: [_ TRUE] -> w175
            frame Default {
              n65 = Delete From Array(array=w183) -> (deleted portion=w179:T5, array with subset deleted=w182:T6)  [unwired: 2 in]
              n66 = Build Array (concatenate)(w181, w179) -> (w180:T6)
            }
            frame "GroupL" {
              # "Remove Left Token"
              n67 = Delete From Array(array=w185) -> (array with subset deleted=w184:T6)  [unwired: 2 in, 1 out]
            }
          }
          n68 = Empty Array?(array=w169) -> (empty?=w167:bool)
          n69 = Or(x=w167, y=w175) -> (x .or. y?=w168:bool)
        }
      }
      frame "Comma" {
        n70 = while {
          shift-right: [w196] -> w191
          shift-left: w192 -> [w193]
          shift-right: [w205] -> w189
          shift-left: w190 -> [w204]
          tunnel: w188 -> [w199]
          stop <- w195 stop-if-true
          n71 = Reverse 1D Array(array=w193) -> (reversed array=w201:T6)
          n72 = Index Array(array=w201) -> (element=w203:T5)  [unwired: 1 in]
          n73 = Unbundle By Name(w203) -> ("Token"=w200:T4)
          n74 = Index Array(array=w199, index=w200) -> (element=w198:T8)
          n75 = Unbundle By Name(w198) -> ("Type"=w197:T9)
          n76 = case shown="\"GroupL\"" w197 {
            tunnel: [w207 w213] -> w205
            tunnel: w204 -> [w208 w213]
            tunnel: [w209 w211] -> w196
            tunnel: w193 -> [w210 w211]
            tunnel: [_ TRUE] -> w202
            frame Default {
              n77 = Delete From Array(array=w210) -> (deleted portion=w206:T5, array with subset deleted=w209:T6)  [unwired: 2 in]
              n78 = Build Array (concatenate)(w208, w206) -> (w207:T6)
            }
            frame "GroupL" {
            }
          }
          n79 = Empty Array?(array=w196) -> (empty?=w194:bool)
          n80 = Or(x=w194, y=w202) -> (x .or. y?=w195:bool)
        }
      }
      frame "Operand" {
        n81 = Build Array (concatenate)(w217, w214) -> (w215:T6)
      }
    }
  }
  n82 = Reverse 1D Array(array=w10) -> (reversed array=w8:T6)
  n83 = Build Array (concatenate)(w11, w8) -> (w5:T6)
  n84 = for {
    tunnel: w5 -> [w219] mode=indexing
    shift-right: [w222] -> w4
    shift-left: dbl[] [] -> [w223]
    tunnel: "String" -> [w220]
    tunnel: "NameSpace" -> [w218]
    n85 = Unbundle By Name(w219) -> ("Token"=w221:T4)
    n86 = case shown="\"LSHIFT\"" w221 {
      tunnel: w223 -> [w232 w244 w259 w271 w276 w283 w290 w298 w306 w314 w322 w330 w331 w338 w347 w359 w371 w380 w389 w399 w406]
      tunnel: [w226 w239 w258 w268 w275 w280 w287 w295 w303 w311 w319 w327 w331 w335 w344 w356 w368 w377 w386 w396 w403] -> w222
      tunnel: w220 -> [w227 w240 w261 _ _ _ _ _ _ _ _ _ _ _ _ _ _ _ _ _ _]
      tunnel: w219 -> [w224 w238 w260 _ _ _ _ _ _ _ _ _ _ _ _ _ _ _ _ _ _]
      tunnel: w218 -> [_ w237 _ _ _ _ _ _ _ _ _ _ _ _ _ _ _ _ _ _ _]
      frame "Dnumeric", "INumeric" {
        n87 = Unbundle By Name(w224) -> ("Start"=w229:i32, "End"=w230:i32)
        n88 = Compound Arithmetic op=ADD(invert w229, w230) -> (w231:i32)
        n89 = String Subset(string=w227, offset (0)=w229, length (rest)=w231) -> (substring=w228:string)
        n90 = Fract/Exp String To Number(string=w228) -> (number=w225:dbl)  [unwired: 3 in, 1 out]
        n91 = Build Array (concatenate)(w232, w225) -> (w226:dbl[])
      }
      frame "Identifier" {
        n92 = Unbundle By Name(w238) -> ("Start"=w241:i32, "End"=w242:i32)
        n93 = Compound Arithmetic op=ADD(invert w241, w242) -> (w243:i32)
        n94 = String Subset(string=w240, offset (0)=w241, length (rest)=w243) -> (substring=w236:string)
        n95 = Get Variant Attribute(Variant=w237, name=w236) -> (value=w234:variant)  [unwired: 2 in, 3 out]
        n96 = call <vilib>:"Get Type Information.vi"("variant"=w234) -> ("type"=w235:T10)  [unwired: 6 in, 4 out]
        n97 = case shown="\"I8\"..\"U64\"" w235 {
          tunnel: w234 -> [_ w250 w253 w256]
          tunnel: [nan w246 w251 w254] -> w233
          frame "Void", Default {
          }
          frame "Boolean" {
            n98 = Variant To Data(type=TRUE, Variant=w250) -> (data=w248:bool)  [unwired: 1 in, 1 out]
            n99 = Boolean To (0,1)(Boolean=w248) -> (0, 1=w247:i16)
            n100 = To Double Precision Float(number=w247) -> (double precision float=w246:dbl)
          }
          frame "Double Float" {
            n101 = Variant To Data(type=0.0, Variant=w253) -> (data=w251:dbl)  [unwired: 1 in, 1 out]
          }
          frame "I8".."U64" {
            n102 = Variant To Data(type=0.0, Variant=w256) -> (data=w254:dbl)  [unwired: 1 in, 1 out]
          }
        }
        n103 = Build Array (concatenate)(w244, w233) -> (w239:dbl[])
      }
      frame "FUNC" {
        n104 = Unbundle By Name(w260) -> ("Start"=w262:i32, "End"=w263:i32)
        n105 = Compound Arithmetic op=ADD(invert w262, w263) -> (w264:i32)
        n106 = String Subset(string=w261, offset (0)=w262, length (rest)=w264) -> (substring=w257:string)
        n107 = call "Functions.vi"("FUNCTION"=w257, "StackIn"=w259) -> ("StackOut"=w258:dbl[])  [unwired: 9 in]
      }
      frame "DIV" {
        n108 = Delete From Array(array=w271) -> (deleted portion=w266:dbl, array with subset deleted=w270:dbl[])  [unwired: 2 in]
        n109 = Delete From Array(array=w270) -> (deleted portion=w267:dbl, array with subset deleted=w269:dbl[])  [unwired: 2 in]
        n110 = Divide(x=w267, y=w266) -> (x/y=w265:dbl)
        n111 = Build Array (concatenate)(w269, w265) -> (w268:dbl[])
      }
      frame "USUB" {
        n112 = Delete From Array(array=w276) -> (deleted portion=w273:dbl, array with subset deleted=w274:dbl[])  [unwired: 2 in]
        n113 = Negate(x=w273) -> (-x=w272:dbl)
        n114 = Build Array (concatenate)(w274, w272) -> (w275:dbl[])
      }
      frame "ADD" {
        n115 = Delete From Array(array=w283) -> (deleted portion=w278:dbl, array with subset deleted=w282:dbl[])  [unwired: 2 in]
        n116 = Delete From Array(array=w282) -> (deleted portion=w279:dbl, array with subset deleted=w281:dbl[])  [unwired: 2 in]
        n117 = Add(x=w279, y=w278) -> (x+y=w277:dbl)
        n118 = Build Array (concatenate)(w281, w277) -> (w280:dbl[])
      }
      frame "EXP" {
        n119 = Delete From Array(array=w290) -> (deleted portion=w284:dbl, array with subset deleted=w289:dbl[])  [unwired: 2 in]
        n120 = Delete From Array(array=w289) -> (deleted portion=w285:dbl, array with subset deleted=w288:dbl[])  [unwired: 2 in]
        n121 = Power Of X(1:w285, 2:w284) -> (0:w286:dbl)
        n122 = Build Array (concatenate)(w288, w286) -> (w287:dbl[])
      }
      frame "GREATER" {
        n123 = Delete From Array(array=w298) -> (deleted portion=w293:dbl, array with subset deleted=w297:dbl[])  [unwired: 2 in]
        n124 = Delete From Array(array=w297) -> (deleted portion=w294:dbl, array with subset deleted=w296:dbl[])  [unwired: 2 in]
        n125 = Greater?(x=w294, y=w293) -> (0:w292:bool)
        n126 = Boolean To (0,1)(Boolean=w292) -> (0, 1=w291:i16)
        n127 = Build Array (concatenate)(w296, w291) -> (w295:dbl[])
      }
      frame "GREATEREQ" {
        n128 = Delete From Array(array=w306) -> (deleted portion=w301:dbl, array with subset deleted=w305:dbl[])  [unwired: 2 in]
        n129 = Delete From Array(array=w305) -> (deleted portion=w302:dbl, array with subset deleted=w304:dbl[])  [unwired: 2 in]
        n130 = Greater Or Equal?(x=w302, y=w301) -> (x >= y?=w300:bool)
        n131 = Boolean To (0,1)(Boolean=w300) -> (0, 1=w299:i16)
        n132 = Build Array (concatenate)(w304, w299) -> (w303:dbl[])
      }
      frame "EQUAL" {
        n133 = Delete From Array(array=w314) -> (deleted portion=w309:dbl, array with subset deleted=w313:dbl[])  [unwired: 2 in]
        n134 = Delete From Array(array=w313) -> (deleted portion=w310:dbl, array with subset deleted=w312:dbl[])  [unwired: 2 in]
        n135 = Equal?(x=w310, y=w309) -> (x = y?=w308:bool)
        n136 = Boolean To (0,1)(Boolean=w308) -> (0, 1=w307:i16)
        n137 = Build Array (concatenate)(w312, w307) -> (w311:dbl[])
      }
      frame "LESS" {
        n138 = Delete From Array(array=w322) -> (deleted portion=w317:dbl, array with subset deleted=w321:dbl[])  [unwired: 2 in]
        n139 = Delete From Array(array=w321) -> (deleted portion=w318:dbl, array with subset deleted=w320:dbl[])  [unwired: 2 in]
        n140 = Less?(x=w318, y=w317) -> (x < y?=w316:bool)
        n141 = Boolean To (0,1)(Boolean=w316) -> (0, 1=w315:i16)
        n142 = Build Array (concatenate)(w320, w315) -> (w319:dbl[])
      }
      frame "LESSEQ" {
        n143 = Delete From Array(array=w330) -> (deleted portion=w325:dbl, array with subset deleted=w329:dbl[])  [unwired: 2 in]
        n144 = Delete From Array(array=w329) -> (deleted portion=w326:dbl, array with subset deleted=w328:dbl[])  [unwired: 2 in]
        n145 = Less Or Equal?(x=w326, y=w325) -> (x <= y?=w324:bool)
        n146 = Boolean To (0,1)(Boolean=w324) -> (0, 1=w323:i16)
        n147 = Build Array (concatenate)(w328, w323) -> (w327:dbl[])
      }
      frame Default {
      }
      frame "SUB" {
        n148 = Delete From Array(array=w338) -> (deleted portion=w333:dbl, array with subset deleted=w337:dbl[])  [unwired: 2 in]
        n149 = Delete From Array(array=w337) -> (deleted portion=w334:dbl, array with subset deleted=w336:dbl[])  [unwired: 2 in]
        n150 = Subtract(x=w334, y=w333) -> (x-y=w332:dbl)
        n151 = Build Array (concatenate)(w336, w332) -> (w335:dbl[])
      }
      frame "LSHIFT" {
        n152 = Delete From Array(array=w347) -> (deleted portion=w342:dbl, array with subset deleted=w346:dbl[])  [unwired: 2 in]
        n153 = To Long Integer(number=w342) -> (32bit integer=w339:i32)
        n154 = Delete From Array(array=w346) -> (deleted portion=w343:dbl, array with subset deleted=w345:dbl[])  [unwired: 2 in]
        n155 = To Long Integer(number=w343) -> (32bit integer=w340:i32)
        n156 = Logical Shift(y=w339, x=w340) -> (x << y=w341:i32)
        n157 = Build Array (concatenate)(w345, w341) -> (w344:dbl[])
      }
      frame "LOGOR" {
        n158 = Delete From Array(array=w359) -> (deleted portion=w354:dbl, array with subset deleted=w358:dbl[])  [unwired: 2 in]
        n159 = To Long Integer(number=w354) -> (32bit integer=w353:i32)
        n160 = Delete From Array(array=w358) -> (deleted portion=w355:dbl, array with subset deleted=w357:dbl[])  [unwired: 2 in]
        n161 = To Long Integer(number=w355) -> (32bit integer=w352:i32)
        n162 = Not Equal To 0?(x=w353) -> (x != 0?=w350:bool)
        n163 = Not Equal To 0?(x=w352) -> (x != 0?=w351:bool)
        n164 = Or(x=w350, y=w351) -> (x .or. y?=w349:bool)
        n165 = Boolean To (0,1)(Boolean=w349) -> (0, 1=w348:i16)
        n166 = Build Array (concatenate)(w357, w348) -> (w356:dbl[])
      }
      frame "LOGAND" {
        n167 = Delete From Array(array=w371) -> (deleted portion=w366:dbl, array with subset deleted=w370:dbl[])  [unwired: 2 in]
        n168 = To Long Integer(number=w366) -> (32bit integer=w365:i32)
        n169 = Delete From Array(array=w370) -> (deleted portion=w367:dbl, array with subset deleted=w369:dbl[])  [unwired: 2 in]
        n170 = To Long Integer(number=w367) -> (32bit integer=w364:i32)
        n171 = Not Equal To 0?(x=w365) -> (x != 0?=w362:bool)
        n172 = Not Equal To 0?(x=w364) -> (x != 0?=w363:bool)
        n173 = And(x=w362, y=w363) -> (x .and. y?=w361:bool)
        n174 = Boolean To (0,1)(Boolean=w361) -> (0, 1=w360:i16)
        n175 = Build Array (concatenate)(w369, w360) -> (w368:dbl[])
      }
      frame "BITOR" {
        n176 = Delete From Array(array=w380) -> (deleted portion=w375:dbl, array with subset deleted=w379:dbl[])  [unwired: 2 in]
        n177 = To Long Integer(number=w375) -> (32bit integer=w373:i32)
        n178 = Delete From Array(array=w379) -> (deleted portion=w376:dbl, array with subset deleted=w378:dbl[])  [unwired: 2 in]
        n179 = To Long Integer(number=w376) -> (32bit integer=w374:i32)
        n180 = Or(x=w373, y=w374) -> (x .or. y?=w372:i32)
        n181 = Build Array (concatenate)(w378, w372) -> (w377:dbl[])
      }
      frame "BITAND" {
        n182 = Delete From Array(array=w389) -> (deleted portion=w384:dbl, array with subset deleted=w388:dbl[])  [unwired: 2 in]
        n183 = To Long Integer(number=w384) -> (32bit integer=w382:i32)
        n184 = Delete From Array(array=w388) -> (deleted portion=w385:dbl, array with subset deleted=w387:dbl[])  [unwired: 2 in]
        n185 = To Long Integer(number=w385) -> (32bit integer=w383:i32)
        n186 = And(x=w382, y=w383) -> (x .and. y?=w381:i32)
        n187 = Build Array (concatenate)(w387, w381) -> (w386:dbl[])
      }
      frame "RSHIFT" {
        n188 = Delete From Array(array=w399) -> (deleted portion=w394:dbl, array with subset deleted=w398:dbl[])  [unwired: 2 in]
        n189 = To Long Integer(number=w394) -> (32bit integer=w391:i32)
        n190 = Delete From Array(array=w398) -> (deleted portion=w395:dbl, array with subset deleted=w397:dbl[])  [unwired: 2 in]
        n191 = To Long Integer(number=w395) -> (32bit integer=w392:i32)
        n192 = Negate(x=w391) -> (-x=w390:i32)
        n193 = Logical Shift(y=w390, x=w392) -> (x << y=w393:i32)
        n194 = Build Array (concatenate)(w397, w393) -> (w396:dbl[])
      }
      frame "MULT" {
        n195 = Delete From Array(array=w406) -> (deleted portion=w401:dbl, array with subset deleted=w405:dbl[])  [unwired: 2 in]
        n196 = Delete From Array(array=w405) -> (deleted portion=w402:dbl, array with subset deleted=w404:dbl[])  [unwired: 2 in]
        n197 = Multiply(x=w402, y=w401) -> (x*y=w400:dbl)
        n198 = Build Array (concatenate)(w404, w400) -> (w403:dbl[])
      }
    }
  }
  n199 = Index Array(array=w4) -> (element=→"element":dbl)  [unwired: 1 in]
